vi "MecaDrivePoseEst_Kalman_H_Callback.vi"(9 "U":T1, 10 "X":T1, 11 "ExtraPassedData":variant) -> (0 "Error":bool, 3 "Result":T1)   [LabVIEW 2019, in "Trajectory_Library.lvlib"]
doc: "Swerve Drive Pose Estimator, Kalman Filter H function. \n\nThis function returns row 2 of the X matrix.\n\nInput:\n - ExtraPassedData -- Variant contaiing extra data for the callback For this function the extra data should be empty..\n - X Matrix -- X matrix\n - U Matrix -- U matrix\n\nOutput:\n - Result -- Matrix resulting from calculation\n - Error -- If TRUE an error occured"
uses:
  <vilib>/Analysis/Matrix/Datatypes/RealMatrix.ctl
  Trajectory_Library.lvlib
  <vilib>/Analysis/Matrix/NI_Matrix.lvlib
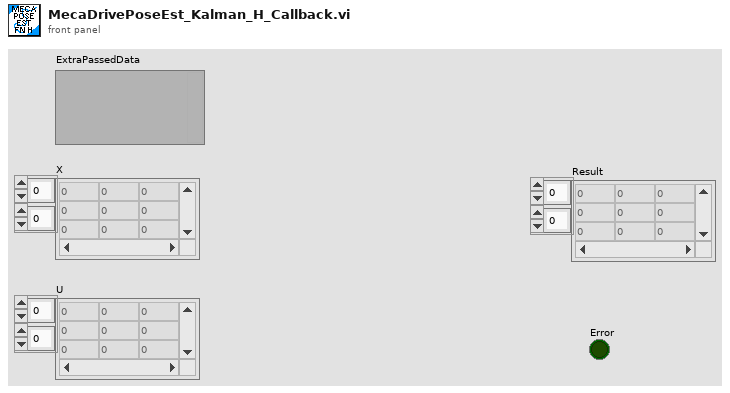
[diagram p1: front panel]
types:
  T1 = typedef "NI_Matrix.lvlib/RealMatrix.ctl" = dbl[][]
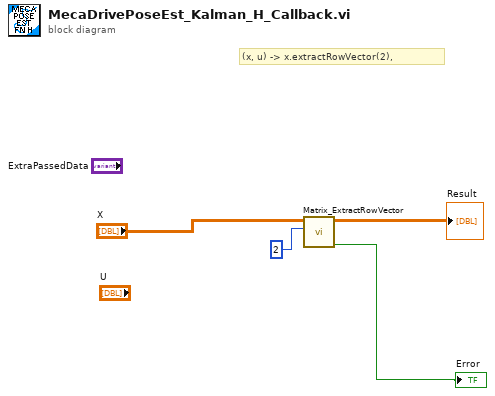
[diagram p0: block diagram]
diagram:
  # "(x, u) -> x.extractRowVector(2),"
  n1 = call "Matrix_ExtractRowVector.vi"("Row"=2, "input matrix"="X") -> ("Error"=→"Error":bool, "output row"=→"Result":T1)  [unwired: 8 in]
